vi "give_monthly_popup.vi"(8 "error in (no error)":errorcluster, 11 "HelioUpdateMH100803 in":refnum<class "HelioUpdateMH100803.lvclass">) -> (0 "error out":errorcluster, 3 "HelioUpdateMH100803 out":refnum<class "HelioUpdateMH100803.lvclass">)   [LabVIEW 2010, in "HelioUpdateMH100803.lvclass"]
uses:
  HelioUpdateMH100803.lvclass
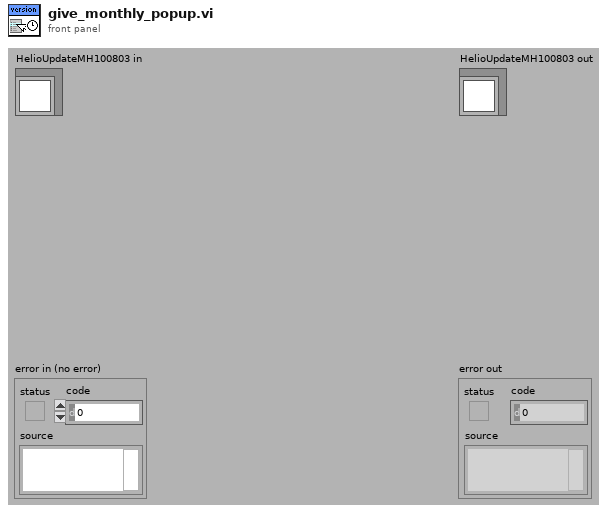
[diagram p1: front panel]
types:
  T1 = enum16{"open", "replace", "create", "open or create", "replace or create", "replace or create with confirmation"}
  T2 = typedef "LVDateTimeRec.ctl" = cluster{"fractional second":dbl, "second":i32, "minute":i32, "hour":i32, "day of month":i32, "month":i32, "year":i32, "day of week":i32, "day of year":i32, "DST":i32}
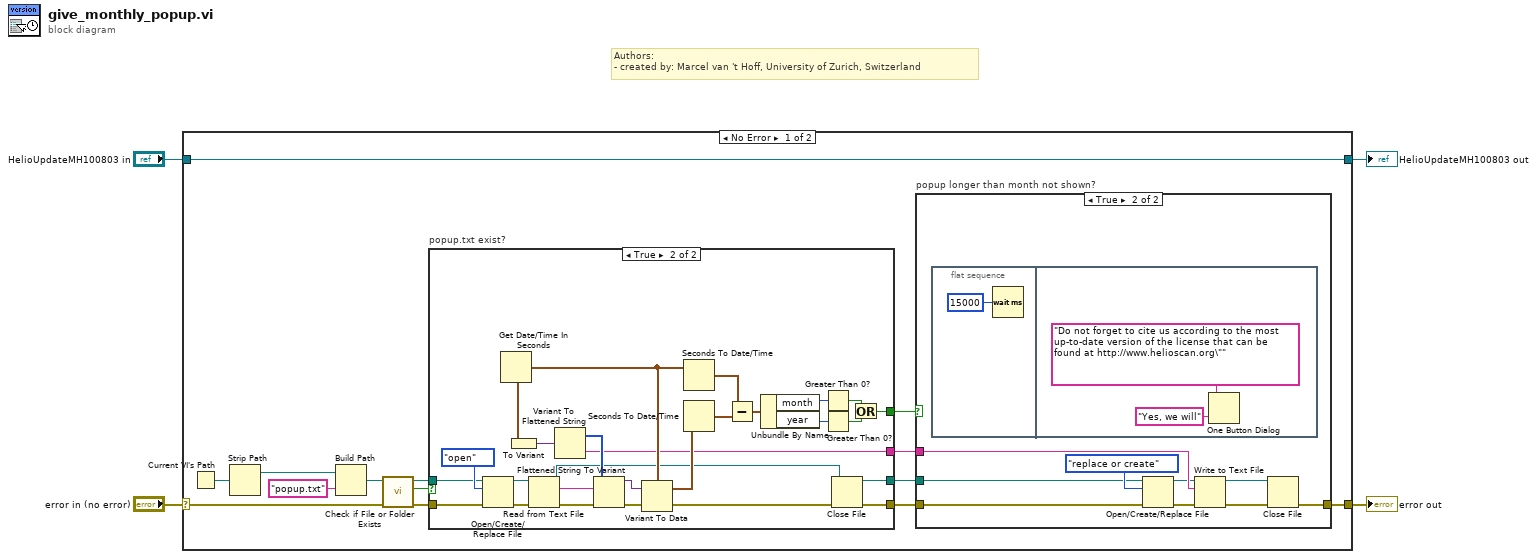
[diagram p0: block diagram]
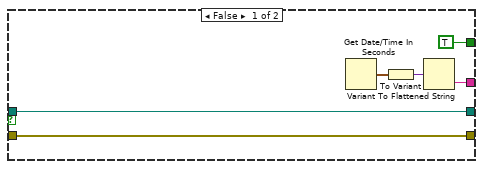
[diagram p2: hidden frame]
diagram:
  # "Authors: \n- created by: Marcel van 't Hoff, University of Zurich, Switzerland"
  n1 = case shown="No Error" "error in (no error)" {
    selector: "error in (no error)" -> [w9 w65]
    tunnel: [w5 w65] -> w3
    tunnel: [w18 w64] -> w1
    tunnel: "HelioUpdateMH100803 in" -> [w18 w64]
    frame No Error {
      n2 = Current VI's Path() -> (path=w17:path)
      n3 = Strip Path(path=w17) -> (stripped path=w16:path)  [unwired: 1 out]
      n4 = Build Path(base path=w16, name or relative path="popup.txt") -> (appended path=w10:path)
      n5 = call <vilib>:"Check if File or Folder Exists.vi"("error in (no error)"=w9, "path"=w10) -> ("error out"=w7:errorcluster, "file or folder exists?"=w6:bool, "dup path"=w8:path)  [unwired: 7 in]
      n6 = case "popup.txt exist?" shown="True" w6 {
        tunnel: [w19 w25] -> w14
        tunnel: [w20 w26] -> w13
        tunnel: [w22 w37] -> w12
        tunnel: [TRUE w33] -> w11
        tunnel: w8 -> [w19 w30]
        tunnel: w7 -> [w20 w29]
        frame False {
          n7 = Get Date/Time In Seconds() -> (seconds since 1Jan1904=w23:timestamp)
          n8 = To Variant(anything=w23) -> (Variant=w24:variant)
          n9 = Variant To Flattened String(Variant=w24) -> (data string=w22:string)  [unwired: 1 out]
        }
        frame True {
          n10 = Open/Create/Replace File(file path (use dialog)=w30, error in=w29, operation (0:open)=T1."open") -> (refnum out=w32:refnum<file>, error out=w31:errorcluster)  [unwired: 3 in, 1 out]
          n11 = Get Date/Time In Seconds() -> (seconds since 1Jan1904=w44:timestamp)
          n12 = To Variant(anything=w44) -> (Variant=w49:variant)
          n13 = Read from Text File(file (use dialog)=w32, error in=w31) -> (refnum out=w28:refnum<file>, text=w46:string, error out=w45:errorcluster)  [unwired: 2 in, 1 out]
          n14 = Variant To Flattened String(Variant=w49) -> (data string=w37:string, 1:w47:i16[])
          n15 = Flattened String To Variant(4:w45, 6:w46, 7:w47) -> (0:w39:errorcluster, 3:w48:variant)
          n16 = Variant To Data(error in=w39, Variant=w48, type=w44) -> (error out=w27:errorcluster, data=w43:timestamp)
          n17 = Seconds To Date/Time(time stamp (now)=w44) -> (date time rec=w42:T2)  [unwired: 1 in]
          n18 = Seconds To Date/Time(time stamp (now)=w43) -> (date time rec=w41:T2)  [unwired: 1 in]
          n19 = Subtract(x=w42, y=w41) -> (x-y=w40:T2)
          n20 = Unbundle By Name(w40) -> ("month"=w38:i32, "year"=w36:i32)
          n21 = Greater Than 0?(x=w38) -> (x > 0?=w35:bool)
          n22 = Greater Than 0?(x=w36) -> (x > 0?=w34:bool)
          n23 = Close File(refnum=w28, error in=w27) -> (path=w25:path, error out=w26:errorcluster)
          n24 = Or(x=w35, y=w34) -> (x .or. y?=w33:bool)
        }
      }
      n25 = case "popup longer than month not shown?" shown="True" w11 {
        tunnel: w14 -> [_ w56]
        tunnel: w13 -> [w51 w55]
        tunnel: [w51 w52] -> w5
        tunnel: w12 -> [_ w60]
        frame False {
        }
        frame True {
          n26 = flat-sequence {
            frame #0 {
              n27 = Wait (ms)(milliseconds to wait=u32 15000) -> ()  [unwired: 1 out]
            }
            frame #1 {
              n28 = One Button Dialog(message="Do not forget to cite us according to the most up-to-date version of the license that can be found at http://www.helioscan.org\"", button name ("OK")="Yes, we will") -> ()  [unwired: 1 out]
            }
          }
          n29 = Open/Create/Replace File(file path (use dialog)=w56, error in=w55, operation (0:open)=T1."replace or create") -> (refnum out=w59:refnum<file>, error out=w57:errorcluster)  [unwired: 3 in, 1 out]
          n30 = Write to Text File(file (use dialog)=w59, text=w60, error in=w57) -> (refnum out=w53:refnum<file>, error out=w54:errorcluster)  [unwired: 1 in, 1 out]
          n31 = Close File(refnum=w53, error in=w54) -> (error out=w52:errorcluster)  [unwired: 1 out]
        }
      }
    }
    frame Error {
    }
  }
  "error out" <- w3
  "HelioUpdateMH100803 out" <- w1
